vi "Reset Scintillators.vi"(8 "error in (no error)":errorcluster, 10 "No hit color":T1, 11 "Scintillator plane in":refnum<vi>) -> (0 "error out":errorcluster, 3 "Scintillator plane out":refnum<vi>)   [LabVIEW 2016]
uses:
  <vilib>/Utility/miscctls.llb/LVRGBAColorTypeDef.ctl
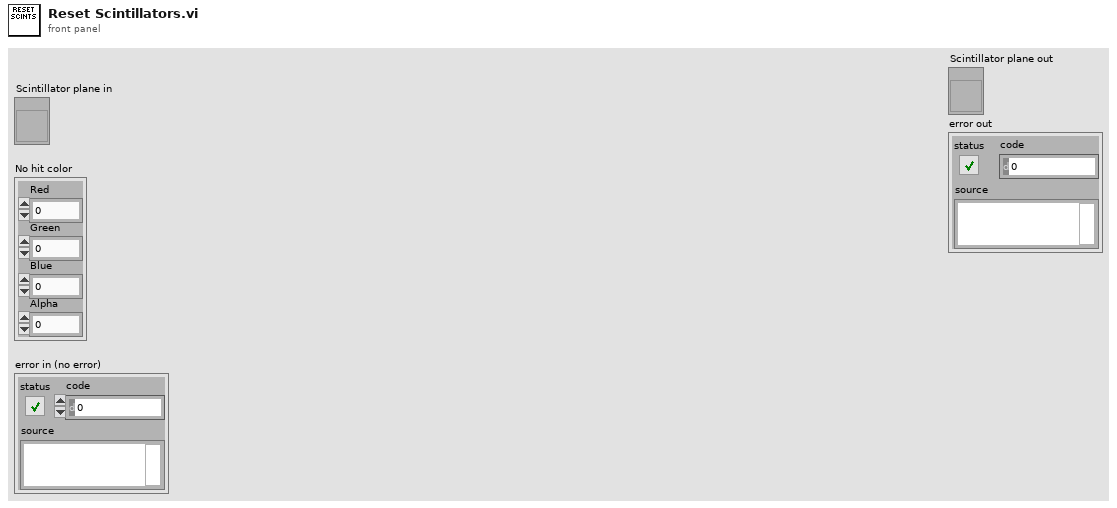
[diagram p1: front panel]
types:
  T1 = typedef "LVRGBAColorTypeDef.ctl" = cluster{"Red":sgl, "Green":sgl, "Blue":sgl, "Alpha":sgl}
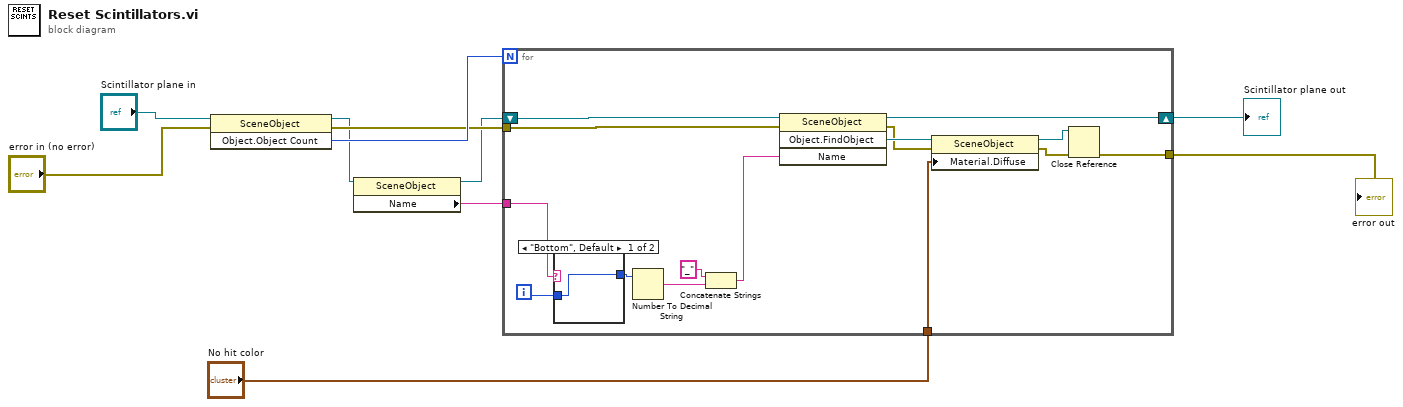
[diagram p0: block diagram]
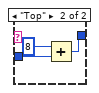
[diagram p2: hidden frame]
diagram:
  n1 = invoke class="SceneObject" method="Object.Object Count"(reference="Scintillator plane in", error in="error in (no error)") -> (reference out=w3:refnum<vi>, error out=w8:errorcluster, "Child Count"=w9:i32)  [unwired: 1 in]
  n2 = property class="SceneObject"(reference=w3) -> (reference out=w2:refnum<vi>, "Name"=w1:string)  [unwired: 1 in, 1 out]
  n3 = for {
    N: w9 -> [_]
    tunnel: w8 -> [w24]
    tunnel: "No hit color" -> [w22]
    tunnel: [w17] -> w4
    shift-right: [w20] -> w6
    shift-left: w2 -> [w25]
    tunnel: w1 -> [w13]
    i -> [w12]
    n4 = case shown="\"Bottom\", Default" w13 {
      tunnel: w12 -> [w26 w29]
      tunnel: [w26 w28] -> w11
      frame "Bottom", Default {
      }
      frame "Top" {
        n5 = Add(x=8, y=w29) -> (x+y=w28:i32)
      }
    }
    n6 = Number To Decimal String(number=w11) -> (decimal integer string=w16:string)  [unwired: 1 in]
    n7 = Concatenate Strings("_" ("string"), w16) -> (w14:string)
    n8 = invoke class="SceneObject" method="Object.FindObject"(reference=w25, error in=w24, "Name"=w14) -> (reference out=w20:refnum<vi>, error out=w21:errorcluster, "FindObject"=w23:refnum<vi>)  [unwired: 1 in, 1 out]
    n9 = property class="SceneObject"(reference=w23, error in=w21, "Material.Diffuse"=w22) -> (reference out=w18:refnum<vi>, error out=w19:errorcluster)
    n10 = Close Reference(reference=w18, error in (no error)=w19) -> (error out=w17:errorcluster)
  }
  "Scintillator plane out" <- w6
  "error out" <- w4
